vi "Create.vi"(10 "Task ID":string) -> (3 "TaskIdentity out":refnum<class "TaskIdentity.lvclass">)   [LabVIEW 2020, in "Volatus.lvlib" / "TaskIdentity.lvclass"]
uses:
  TaskIdentity.lvclass
  TaskIdentity.lvclass/TaskIdentity.ctl
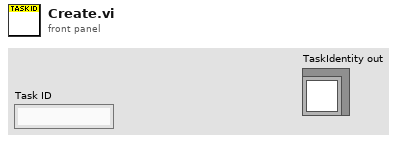
[diagram p1: front panel]
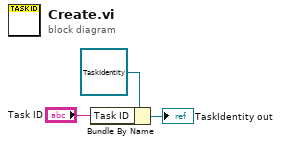
[diagram p0: block diagram]
diagram:
  n1 = Bundle By Name(cluster=refnum<class "TaskIdentity.lvclass"> refnum ("TaskIdentity in"), "Task ID"="Task ID") -> (→"TaskIdentity out":refnum<class "TaskIdentity.lvclass">)
